vi "AVS_Unremote.vi"() -> (11 "VISA session":refnum<visa-resource-name>="GPIB0::20::INSTR")   [LabVIEW 2016]
uses:
  Instrument_Setup_v2.vi
panel:
  out "T (K) 2":dbl=0.00957168277075326 format="%^.3e"
  out "T (K)":dbl=0.00957168277075326 format="%^.3e"
  out "Widerstand":dbl format="%.2f"
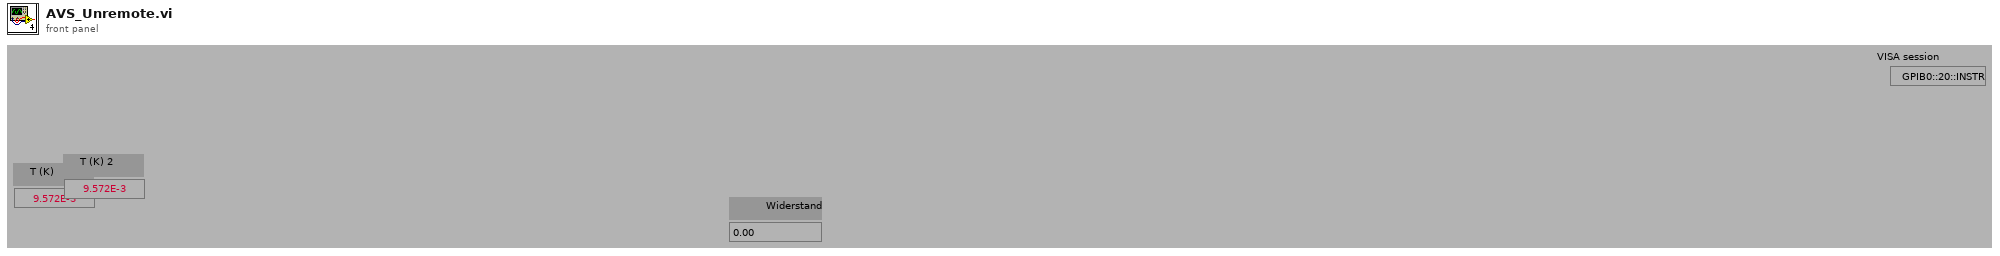
[diagram p1: front panel]
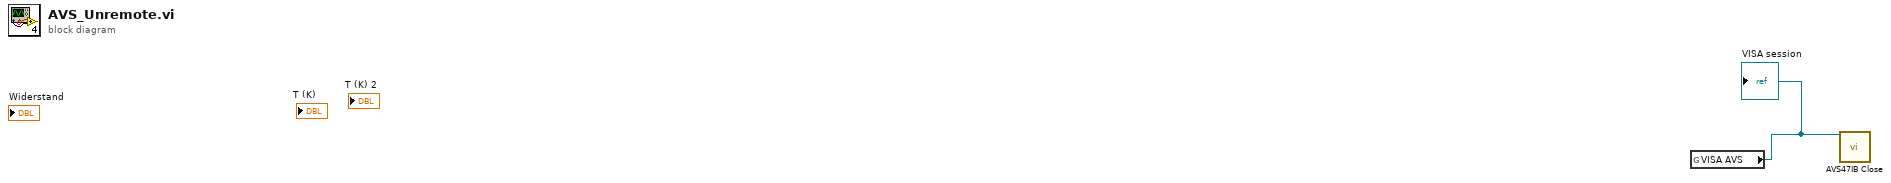
[diagram p0: block diagram]
diagram:
  n1 = global read "Instrument_Setup_v2.vi" "VISA AVS"() -> (w1:refnum<visa-resource-name>)
  "VISA session" <- w1
  n2 = call "AVS47IB Close.vi"("VISA session"=w1) -> ()  [unwired: 14 in, 1 out]
